vi "Teleop.vi"(8 "HARDWARE cluster":T1={"DRIVE MOTORS"=[], "Controller"=[], "ENCODERS"=[], "GYRO HARDWARE"={"Descr"="GYRO", "Installed?"=FALSE, "SPI Bus"=enum."SPI On-Board, CS0", "AnalogChannel"=enum."AI 0", "Calibrate On Open"=TRUE, "Calibrated Center Voltage"=0.0, "Calibration Time (s)"=2.0, "Sample Rate (Hz)"=100.0, "RefName"="", "stack name"="GYRO"}, "AIR"={"PRESSURE"=[], "COMPRESSOR"={"Descr"="COMPRESSOR", "Installed?"=TRUE, "Pneumatics Control Module"=0, "RefName"="COMPRESSOR", "stack name"="COMPRESSOR"}, "SOLENOIDS"=[]}, "MOTORS"=[], "SERVOS"=[], "SONAR"=[], "RELAY"=[], "LIMIT"=[]} {"MOTORS"."Motor Controller" items=["SPARK", "Existing", "SD540", "TALON SRX", "VICTOR SP", "TALON SR", "JAGUAR", "VICTOR"]; "AIR"."PRESSURE"."warning HIGH" format="%.2f"; "AIR"."PRESSURE"."warning LOW" format="%.2f"; "AIR"."PRESSURE"."nominal value" format="%.2f"; "DRIVE MOTORS"."Motor Controller" items=["SPARK", "Existing", "SD540", "TALON SRX", "VICTOR SP", "TALON SR", "JAGUAR", "VICTOR"]; "Controller"."Parameters"."DEADBAND" format="%#_13g"; "Controller"."Parameters"."MIN SPEED" format="%#_13g"; "Controller"."Parameters"."MAX LIMIT" format="%#_13g"}, 10 "Match Info":T29={"Autonomous Elapsed Seconds"=0.0, "TeleOp Elapsed Seconds"=0.0, "Disabled Elapsed Seconds"=0.0, "Visited Autonomous"=FALSE, "Visited TeleOp"=FALSE, "Visited Disabled"=FALSE, "Autonomous Settings"={"Autonomous Style"=enum."Independent", "VI Refnum"=refnum}}, 11 "Call Context":T30) -> ()   [LabVIEW 2017]
doc: "This VI is called for each TeleOp packet received from the DS where the robot is not disabled. It is often used to read from the joysticks and update I/O or to update setpoints for timed control loops. It should complete and return within 20 milliseconds or it may miss DS packets."
uses:
  <vilib>/Rock Robotics/WPI/DriverStation/WPI_DriverStationDerivedRobotMode.ctl
  <vilib>/Rock Robotics/WPI/DriverStation/WPI_DriverStationMatch Info.ctl
  Controls/def HARDWARE CTRL info.ctl
  Controls/def MOTOR info.ctl
  Controls/ctrl MOTOR CTRLR SELECT.ctl
  <vilib>/Rock Robotics/SystemInterfaces/DIO/FPGA_DIOPWMChannel.ctl
  Controls/def USER CONTROL info.ctl
  <vilib>/Rock Robotics/WPI/Joystick/WPI_JoystickDeviceEnum.ctl
  Controls/def JOYSTICK PARAMETERS.ctl
  Controls/def ENCODER info.ctl
  <vilib>/Rock Robotics/SystemInterfaces/DIO/FPGA_DIOChannel.ctl
  <vilib>/Rock Robotics/WPI/Encoder/WPI_EncoderType.ctl
  Controls/def GYRO info.ctl
  <vilib>/Rock Robotics/SystemInterfaces/spilib/spi_bus.ctl
  Controls/ctrl ANALOG CHANNEL SELECT.ctl
  Controls/def AIR PRESSURE info.ctl
  <vilib>/Rock Robotics/SystemInterfaces/AI/FPGA_AIChannel.ctl
  Controls/def COMPRESSOR info.ctl
  Controls/def SOLENOID info.ctl
  <vilib>/Rock Robotics/WPI/Solenoid/WPI_SolenoidChannel.ctl
  <vilib>/Rock Robotics/WPI/Solenoid/WPI_SolenoidValue.ctl
  Controls/def SERVO info.ctl
  Controls/def SONAR info.ctl
  Controls/ctrl SONAR DEVICE SELECT.ctl
  <vilib>/Rock Robotics/WPI/Ultrasonic/WPI_UltrasonicRangeUnits.ctl
  Controls/def RELAY info.ctl
  <vilib>/Rock Robotics/SystemInterfaces/DIO/FPGA_DIORelayChannel.ctl
  <vilib>/Rock Robotics/WPI/Relay/WPI_RelayDirection.ctl
  <vilib>/Rock Robotics/WPI/Relay/WPI_RelayValue.ctl
  Controls/def LIMIT SWITCH info.ctl
  <vilib>/Rock Robotics/Network Tables/NT Read Boolean.vi
  <vilib>/Rock Robotics/Network Tables/NT Read Number.vi
  <vilib>/Rock Robotics/WPI/Utilities/WPI_GetSetVariantRefNum.vi
  <vilib>/Rock Robotics/Network Tables/NT Write Numeric Array.vi
  <vilib>/Rock Robotics/Network Tables/NT Write Boolean Array.vi
panel:
  out "Sample Slider 0":dbl(slide) scale=0.0..5.0
  out "Sample Boolean 1":bool
  out "Sample Boolean 0":bool
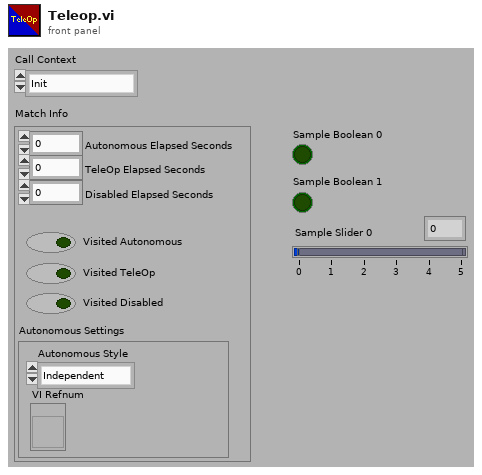
[diagram p1: front panel]
types:
  T1 = typedef "def HARDWARE CTRL info.ctl" = cluster{"DRIVE MOTORS":T2[], "Controller":T5[], "ENCODERS":T8[], "GYRO HARDWARE":T11, "AIR":cluster{"PRESSURE":T14[], "COMPRESSOR":T16, "SOLENOIDS":T17[]}, "MOTORS":T2[], "SERVOS":T20[], "SONAR":T21[], "RELAY":T24[], "LIMIT":T28[]}
  T2 = typedef "def MOTOR info.ctl" = cluster{"Descr":string, "Motor Controller":T3, "PWM ch":T4, "Invert?":bool, "Installed?":bool, "RefName":string, "stack name":string, "remove deadband":bool}
  T3 = typedef "ctrl MOTOR CTRLR SELECT.ctl" = u16
  T4 = typedef "FPGA_DIOPWMChannel.ctl" = enum8{"PWM 0", "PWM 1", "PWM 2", "PWM 3", "PWM 4", "PWM 5", "PWM 6", "PWM 7", "PWM 8", "PWM 9", "PWM MXP 0", "PWM MXP 1", "PWM MXP 2", "PWM MXP 3", "PWM MXP 4", "PWM MXP 5", "PWM MXP 6", "PWM MXP 7", "PWM MXP 8", "PWM MXP 9", "Invalid"}
  T5 = typedef "def USER CONTROL info.ctl" = cluster{"Descr":string, "Installed?":bool, "RefName":string, "JoystickDevice":T6, "Invert Y axis":bool, "Scale":dbl, "AXIS":string, "BUTTONS":string, "POV":string, "Parameters":T7}
  T6 = typedef "WPI_JoystickDeviceEnum.ctl" = enum16{"USB 0", "USB 1", "USB 2", "USB 3", "USB 4", "USB 5"}
  T7 = typedef "def JOYSTICK PARAMETERS.ctl" = cluster{"MAX LIMIT":dbl, "MIN SPEED":dbl, "DEADBAND":dbl, "invert X?":bool, "invert Y?":bool}
  T8 = typedef "def ENCODER info.ctl" = cluster{"Descr":string, "Installed?":bool, "A Channel":T9, "B Channel":T9, "Invert Direction":bool, "Enum":T10, "Gear ratio":dbl, "Cycles per Rev":dbl, "Diameter (in)":dbl[unit], "RefName":string, "stack name":string, "min rate (hz)":dbl, "Samples":u8, "STACK subnames":cluster{"RESET name":string, "STOPPED name":string, "DIRECTION name":string, "RATE name":string, "INSTALLED name":string}}
  T9 = typedef "FPGA_DIOChannel.ctl" = enum8{"DIO 0", "DIO 1", "DIO 2", "DIO 3", "DIO 4", "DIO 5", "DIO 6", "DIO 7", "DIO 8", "DIO 9", "DIO MXP 0", "DIO MXP 1", "DIO MXP 2", "DIO MXP 3", "DIO MXP 4", "DIO MXP 5", "DIO MXP 6", "DIO MXP 7", "DIO MXP 8", "DIO MXP 9", "DIO MXP 10", "DIO MXP 11", "DIO MXP 12", "DIO MXP 13", "DIO MXP 14", "DIO MXP 15", "SPI Port CS1", "SPI Port CS2", "SPI Port CS3", "SPI Port MISO", "SPI Port MOSI", "Invalid"}
  T10 = typedef "WPI_EncoderType.ctl" = enum16{"1x", "2x", "4x"}
  T11 = typedef "def GYRO info.ctl" = cluster{"Descr":string, "Installed?":bool, "SPI Bus":T12, "AnalogChannel":T13, "Calibrate On Open":bool, "Calibrated Center Voltage":dbl, "Calibration Time (s)":dbl, "Sample Rate (Hz)":dbl, "RefName":string, "stack name":string}
  T12 = typedef "spi_bus.ctl" = enum16{"SPI On-Board, CS0", "SPI On-Board, CS1", "SPI On-Board, CS2", "SPI On-Board, CS3", "SPI MXP", "Invalid"}
  T13 = typedef "ctrl ANALOG CHANNEL SELECT.ctl" = enum8{"AI 0", "AI 1", "Invalid"}
  T14 = typedef "def AIR PRESSURE info.ctl" = cluster{"Descr":string, "Installed?":bool, "Channel":T15, "RefName":string, "stack name":string, "MULTIPLIER":dbl, "OFFSET":dbl, "nominal value":dbl, "warning LOW":dbl, "warning HIGH":dbl}
  T15 = typedef "FPGA_AIChannel.ctl" = enum8{"AI 0", "AI 1", "AI 2", "AI 3", "AI MXP 0", "AI MXP 1", "AI MXP 2", "AI MXP 3", "Invalid"}
  T16 = typedef "def COMPRESSOR info.ctl" = cluster{"Descr":string, "Installed?":bool, "Pneumatics Control Module":u8, "RefName":string, "stack name":string}
  T17 = typedef "def SOLENOID info.ctl" = cluster{"Descr":string, "Installed?":bool, "Pneumatics Control Module (0)":u8, "DBL":bool, "SolenoidChannel":T18, "SolenoidChannel":T18, "Default SET":T19, "RefName":string, "Value":string}
  T18 = typedef "WPI_SolenoidChannel.ctl" = enum8{"Solenoid 0", "Solenoid 1", "Solenoid 2", "Solenoid 3", "Solenoid 4", "Solenoid 5", "Solenoid 6", "Solenoid 7", "Invalid"}
  T19 = typedef "WPI_SolenoidValue.ctl" = enum16{"Off", "On", "Forward", "Reverse"}
  T20 = typedef "def SERVO info.ctl" = cluster{"Descr":string, "PWM ch":T4, "Installed?":bool, "Angular range":dbl, "RefName":string, "stack name":string}
  T21 = typedef "def SONAR info.ctl" = cluster{"Descr":string, "Installed?":bool, "Device type":T22, "PING Channel":T9, "ECHO Channel":T9, "RefName":string, "stack name":string, "Samples":i32, "Range Units":T23}
  T22 = typedef "ctrl SONAR DEVICE SELECT.ctl" = enum16{"SRF04 Digital", "MB1010 Digital", "MB1010 Analog", "SRF08 Digital"}
  T23 = typedef "WPI_UltrasonicRangeUnits.ctl" = enum16{"inches", "mm"}
  T24 = typedef "def RELAY info.ctl" = cluster{"Descr":string, "Installed?":bool, "RelayChannel":T25, "Relay Direction":T26, "Relay Value":T27, "RefName":string, "Value":string}
  T25 = typedef "FPGA_DIORelayChannel.ctl" = enum8{"Relay 0", "Relay 1", "Relay 2", "Relay 3", "Invalid"}
  T26 = typedef "WPI_RelayDirection.ctl" = enum16{"Both directions", "Forward only", "Reverse only"}
  T27 = typedef "WPI_RelayValue.ctl" = enum16{"Off", "On", "Forward", "Reverse"}
  T28 = typedef "def LIMIT SWITCH info.ctl" = cluster{"Descr":string, "Installed?":bool, "A Channel":T9, "Normally Closed?":bool, "RefName":string, "stack name":string}
  T29 = typedef "WPI_DriverStationMatch Info.ctl" = cluster{"Autonomous Elapsed Seconds":dbl, "TeleOp Elapsed Seconds":dbl, "Disabled Elapsed Seconds":dbl, "Visited Autonomous":bool, "Visited TeleOp":bool, "Visited Disabled":bool, "Autonomous Settings":cluster{"Autonomous Style":enum16{"Iterative", "Independent"}, "VI Refnum":refnum<vi>}}
  T30 = typedef "WPI_DriverStationDerivedRobotMode.ctl" = enum16{"Init", "Execute", "Stop"}
  T31 = typedef "WPI_JoystickDevRef.ctl" = cluster{"Device":T6}
  T32 = typedef "WPI_RobotDriveDevRef.ctl" = cluster{"DevStatus":errorcluster, "Motors[]":T33[], "Square Inputs":bool, "Max Output":dbl}
  T33 = typedef "WPI_MotorControlDeviceRef.ctl" = cluster{"DeviceStatus":errorcluster, "Type":T34, "PWM":cluster{"PWM Channel":T4, "DeadBand":T35}, "CAN":cluster{"Device Number":u8, "SetOutput VI Ref":variant, "GetOutput VI Ref":variant, "Enable VI Ref":variant, "Disable VI Ref":variant, "Data":variant}, "Invert":bool, "DIO PWM":cluster{"PWM \"Enable\" Channel":T4, "DIO Channel":T9, "PWM Rate":dbl}}
  T34 = typedef "WPI_MotorControlType.ctl" = enum16{"PWM", "CAN", "DIO PWM"}
  T35 = typedef "WPI_PWMDeadband.ctl" = cluster{"Name":string, "maxPositivePwm":i32, "minPositivePwm":i32, "centerPwm":i32, "maxNegativePwm":i32, "minNegativePwm":i32, "angularRange":u16}
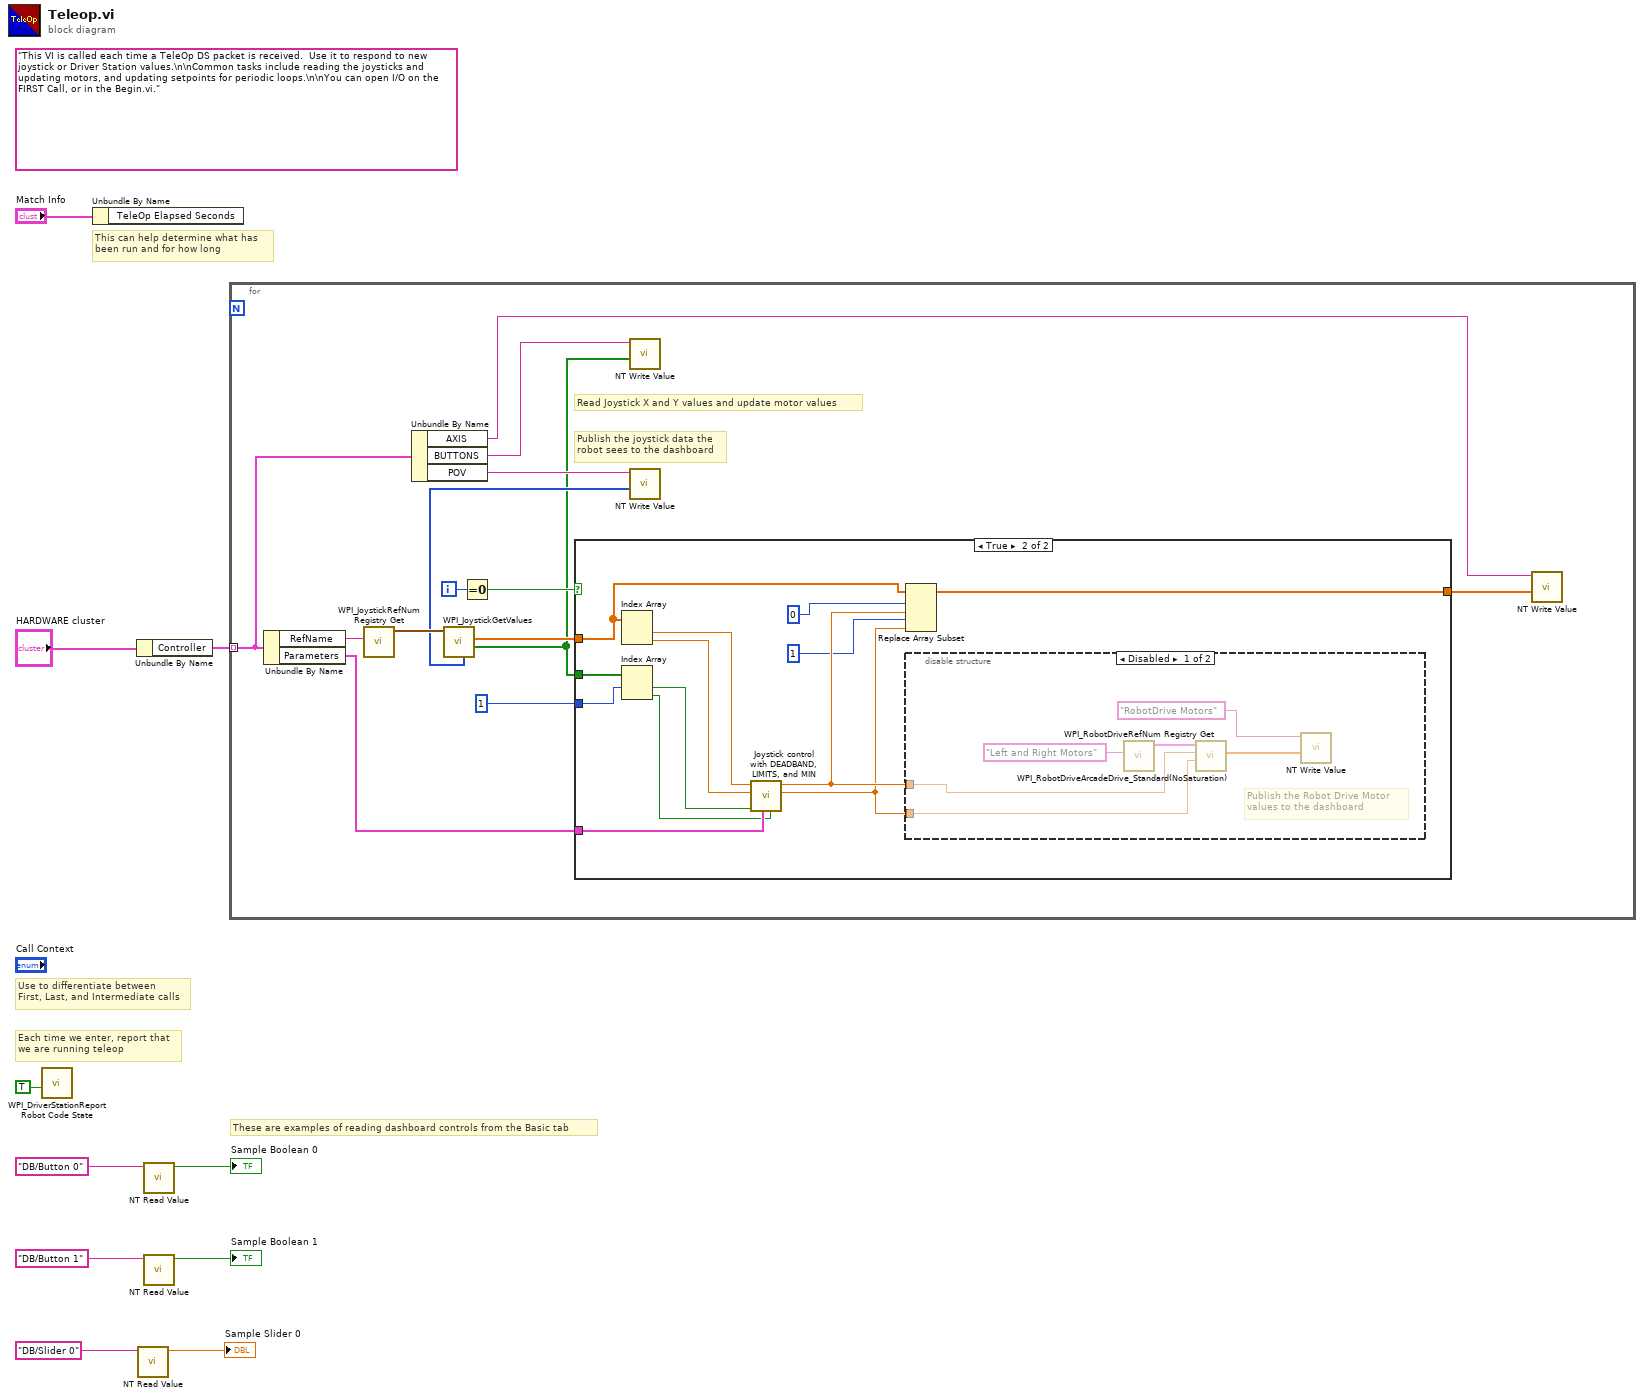
[diagram p0: block diagram]
diagram:
  (unwired) "This VI is called each time a TeleOp DS packet is received.  Use it to respond to new joystick or Driver Station values.\n\nCommon tasks include reading the joysticks and updating motors, and updating setpoints for periodic loops.\n\nYou can open I/O on the FIRST Call, or in the Begin.vi."
  # "These are examples of reading dashboard controls from the Basic tab"
  # "Each time we enter, report that\nwe are running teleop"
  # "Use to differentiate between\nFirst, Last, and Intermediate calls"
  # "This can help determine what has\nbeen run and for how long"
  n1 = call <vilib>:"WPI_DriverStationReport Robot Code State.vi"("TeleOp"=TRUE ("Autonomous")) -> ()  [unwired: 10 in, 1 out]
  n2 = Unbundle By Name("Match Info") -> ()  [unwired: 1 out]
  n3 = Unbundle By Name("HARDWARE cluster") -> ("Controller"=w1:T5[])
  n4 = call-poly <vilib>:"NT Read Value.vi"("Name"="DB/Slider 0" ("refnum name")) -> ("Numeric"=→"Sample Slider 0":dbl)  [unwired: 9 in, 1 out]
  n5 = call-poly <vilib>:"NT Read Value.vi"("Name"="DB/Button 0" ("refnum name")) -> ("Boolean"=→"Sample Boolean 0":bool)  [unwired: 9 in, 1 out]
  n6 = call-poly <vilib>:"NT Read Value.vi"("Name"="DB/Button 1" ("refnum name")) -> ("Boolean"=→"Sample Boolean 1":bool)  [unwired: 9 in, 1 out]
  n7 = for {
    tunnel: w1 -> [w15] mode=indexing
    i -> [w13]
    # "Publish the joystick data the\nrobot sees to the dashboard"
    # "Read Joystick X and Y values and update motor values"
    n8 = Unbundle By Name(w15) -> ("RefName"=w16:string, "Parameters"=w23:T7)
    n9 = call <vilib>:"WPI_JoystickRefNum Registry Get.vi"("refnum name"=w16) -> ("JoystickDevRef"=w24:T31)  [unwired: 1 in, 9 out]
    n10 = Unbundle By Name(w15) -> ("AXIS"=w20:string, "BUTTONS"=w19:string, "POV"=w17:string)
    n11 = call <vilib>:"WPI_JoystickGetValues.vi"("JoystickDevRef"=w24) -> ("Buttons"=w12:bool[], "Axes"=w22:dbl[], "POVs"=w18:i16[])  [unwired: 6 in, 2 out]
    n12 = Equal To 0?(x=w13) -> (x = 0?=w14:bool)
    n13 = case shown="True" w14 {
      tunnel: w23 -> [_ w38]
      tunnel: w22 -> [w25 w32]
      tunnel: [w25 w33] -> w21
      tunnel: w12 -> [_ w29]
      tunnel: 1 ("index") -> [_ w28]
      frame False {
      }
      frame True {
        n14 = Index Array(array=w32) -> (element #1=w31:dbl, element #2=w30:dbl)  [unwired: 2 in]
        n15 = Index Array(array=w29, index #1=w28) -> (element #1=w27:bool, element #2=w26:bool)  [unwired: 1 in]
        n16 = call "Joystick control with DEADBAND, LIMITS, and MIN.vi"("slow?"=w26, "Parameters"=w38, "TURBO?"=w27, "Joystick Y"=w30, "Joystick X"=w31) -> ("Y out"=w36:dbl, "X out"=w37:dbl)  [unwired: 4 in, 1 out]
        n17 = Replace Array Subset(array=w32, new element #1=w37, index #1=0 ("index"), new element #2=w36, index #2=1 ("index")) -> (w33:dbl[])
        n18 = disable-structure shown="Disabled" {
          disable-tunnel: w37 -> [w40 _]
          disable-tunnel: w36 -> [w39 _]
          frame Disabled {
            # "Publish the Robot Drive Motor\nvalues to the dashboard"
            n19 = call <vilib>:"WPI_RobotDriveRefNum Registry Get.vi"("refnum name"="Left and Right Motors") -> ("RobotDriveDevRef"=w43:T32)  [unwired: 1 in, 9 out]
            n20 = call <vilib>:"WPI_RobotDriveArcadeDrive_Standard(NoSaturation).vi"("Y axis value"=w39, "X axis value"=w40, "RobotDriveDevRef"=w43) -> ("Motor Values"=w42:dbl[])  [unwired: 1 in, 7 out]
            n21 = call-poly <vilib>:"NT Write Value.vi"("Numeric Array"=w42, "Name"="RobotDrive Motors") -> ()  [unwired: 9 in, 1 out]
          }
          frame Enabled {
          }
        }
      }
    }
    n22 = call-poly <vilib>:"NT Write Value.vi"("Boolean Array"=w12, "Name"=w19) -> ()  [unwired: 9 in, 1 out]
    n23 = call-poly <vilib>:"NT Write Value.vi"("Numeric Array"=w18, "Name"=w17) -> ()  [unwired: 9 in, 1 out]
    n24 = call-poly <vilib>:"NT Write Value.vi"("Numeric Array"=w21, "Name"=w20) -> ()  [unwired: 9 in, 1 out]
  }
